vi "DetermineCommandLineArgs.vi"(10 "CLI Arguments":string[](array[string]), 11 "App.Args in":string[](array[string])) -> (3 "App.Args out":string[](array[string]))   [LabVIEW 2019, in "SolutionBuilder.lvlib"]
uses:
  SolutionBuilder/SolutionBuilder.lvlib
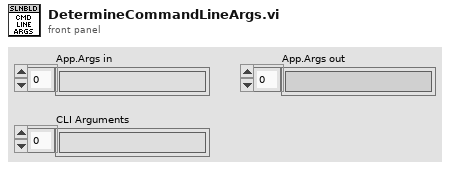
[diagram p1: front panel]
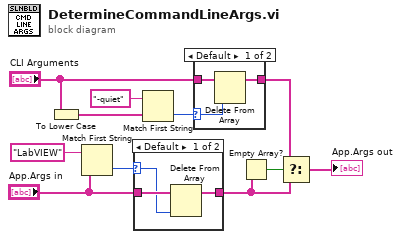
[diagram p0: block diagram]
diagram:
  n1 = To Lower Case(string="CLI Arguments") -> (all lower case string=w4:string[])
  n2 = Match First String(2:"App.Args in", 3:"LabVIEW" ("string")) -> (0:w10:i32)  [unwired: 1 out]
  n3 = case shown="Default" w10 {
    selector: w10 -> [w13 _]
    tunnel: "App.Args in" -> [w14 w15]
    tunnel: [w12 w15] -> w7
    frame Default {
      n4 = Delete From Array(array=w14, index=w13) -> (array with subset deleted=w12:string[])  [unwired: 1 in, 1 out]
    }
    frame -1 {
    }
  }
  n5 = Match First String(2:w4, 3:"-quiet" ("string")) -> (0:w3:i32)  [unwired: 1 out]
  n6 = case shown="Default" w3 {
    selector: w3 -> [w17 _]
    tunnel: "CLI Arguments" -> [w18 w19]
    tunnel: [w16 w19] -> w1
    frame Default {
      n7 = Delete From Array(array=w18, index=w17) -> (array with subset deleted=w16:string[])  [unwired: 1 in, 1 out]
    }
    frame -1 {
    }
  }
  n8 = Empty Array?(array=w7) -> (empty?=w8:bool)
  n9 = Select(t=w1, s=w8, f=w7) -> (s? t:f=→"App.Args out":string[])
